vi "Location to Grpc Device.vi"(10 "Grpc Device Location":T2, 11 "Session Name":string) -> (3 "gRPC Device Options":T1={"session name"="", "address (localhost)"="localhost", "port (31763)"=31763})   [LabVIEW 2020, in "Measurement Service Helpers.lvlib"]
uses:
  Measurement Service Helpers.lvlib
  <vilib>/MeasurementLink/MeasurementLink Discovery Client/RPC Messages/ni_measurementlink_discovery_v1_ServiceLocation.ctl
  gRPC Device Options.ctl
  <vilib>/MeasurementLink/MeasurementLink Discovery Client/MeasurementLink Discovery Client.lvlib
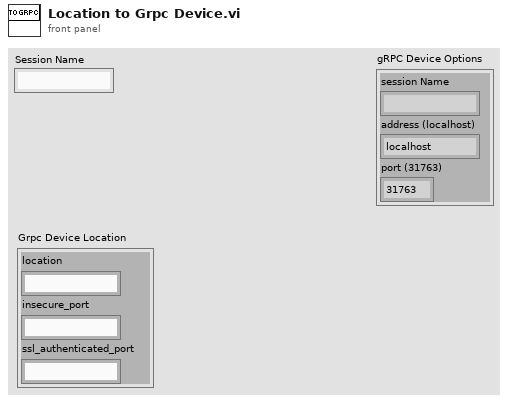
[diagram p1: front panel]
types:
  T1 = typedef "Measurement Service Helpers.lvlib/gRPC Device Options.ctl" = cluster{"session name":string, "address (localhost)":string, "port (31763)":u32}
  T2 = typedef "MeasurementLink Discovery Client.lvlib/ni_measurementlink_discovery_v1_ServiceLocation.ctl" = cluster{"location":string, "insecure_port":string, "ssl_authenticated_port":string}
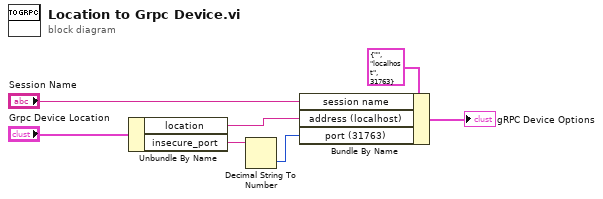
[diagram p0: block diagram]
diagram:
  n1 = Unbundle By Name("Grpc Device Location") -> ("location"=w4:string, "insecure_port"=w3:string)
  n2 = Decimal String To Number(string=w3) -> (number=w6:i32)  [unwired: 2 in, 1 out]
  n3 = Bundle By Name(cluster=T1 {"session name"="", "address (localhost)"="localhost", "port (31763)"=31763} ("NI gRPC Device Server"), "session name"="Session Name", "address (localhost)"=w4, "port (31763)"=w6) -> (→"gRPC Device Options":T1)
